vi "ReadPortsHeader.vi"(0 "data":string) -> (1 "Numbers":i32[](array[numeric]), 2 "Names":string[](array[string]))   [LabVIEW 2009]
panel:
  out "array":string[][](array[string])
  out "after substring":string
  out "subarray":string[](array[string])
  out "subarray 2":string[](array[string])
  out "array w/ subset deleted":string[](array[string])
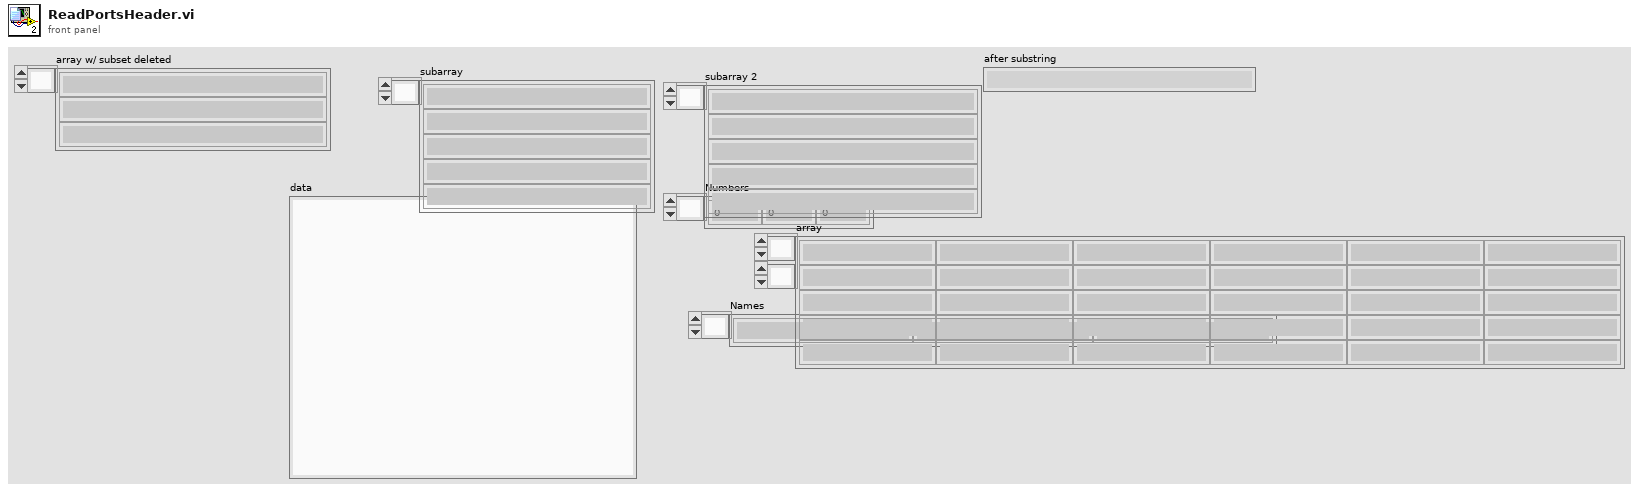
[diagram p1: front panel]
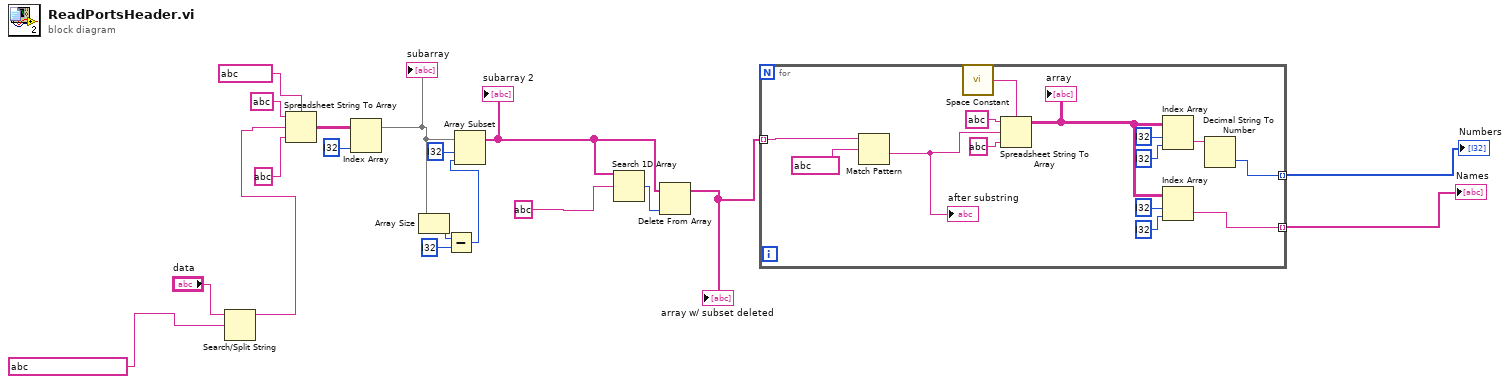
[diagram p0: block diagram]
diagram:
  n1 = Search/Split String(string="data", search string/char (-)=string ? ("regular expression")) -> (substring before match=w3:string)  [unwired: 1 in, 2 out]
  n2 = Spreadsheet String To Array(delimiter (Tab)=string ?, format string=string ?, spreadsheet string=w3, array type (2D Dbl)=string ? ("delimiter (Tab)")) -> (array=w10:string[][])
  n3 = Index Array(array=w10, index (col)=i32 ? ("index (row)")) -> (element=w7:string[])  [unwired: 1 in]
  "subarray" <- w7
  n4 = Array Size(array=w7) -> (size(s)=w6:i32)
  n5 = Subtract(x=w6, y=i32 ?) -> (x-y=w5:i32)
  n6 = Array Subset(array=w7, index=i32 ?, length=w5) -> (w14:string[])
  "subarray 2" <- w14
  n7 = Search 1D Array(1D array=w14, element=string ?) -> (index of element=w15:i32)  [unwired: 1 in]
  n8 = Delete From Array(array=w14, index=w15) -> (array with subset deleted=w17:string[])  [unwired: 1 in, 1 out]
  "array w/ subset deleted" <- w17
  n9 = for {
    tunnel: w17 -> [w23] mode=indexing
    tunnel: [w28] -> w2 mode=indexing
    tunnel: [w24] -> w1 mode=indexing
    n10 = Match Pattern(string=w23, regular expression=string ? ("delimiter (Tab)")) -> (after substring=w21:string)  [unwired: 1 in, 3 out]
    "after substring" <- w21
    n11 = call <vilib>:"Space Constant.vi"() -> ("String"=w20:string)
    n12 = Spreadsheet String To Array(delimiter (Tab)=w20, format string=string ?, spreadsheet string=w21, array type (2D Dbl)=string ? ("delimiter (Tab)")) -> (array=w25:string[][])
    "array" <- w25
    n13 = Index Array(array=w25, index (row)=i32 ?, index (col)=i32 ? ("disabled index (col)")) -> (element=w29:string)
    n14 = Index Array(array=w25, index (row)=i32 ?, index (col)=i32 ? ("disabled index (col)")) -> (element=w24:string)
    n15 = Decimal String To Number(string=w29) -> (number=w28:i32)  [unwired: 2 in, 1 out]
  }
  "Numbers" <- w2
  "Names" <- w1
